vi "ExecuteSkill.vi"(0 "object in":refnum<class "GoToTargetPositionSkill.lvclass">, 2 "Robot in":refnum<class "Robot.lvclass">, 4 "GameRef":refnum<data-value>, 5 "error in (no error)":errorcluster) -> (14 "object out":refnum<class "GoToTargetPositionSkill.lvclass">, 16 "Robot out":refnum<class "Robot.lvclass">, 19 "error out":errorcluster)   [LabVIEW 2023, in "GoToTargetPositionSkill.lvclass"]
uses:
  GoToTargetPositionSkill.lvclass
  Robot_class/Robot.lvclass
  Game_class/Game.lvclass
  Ball_class/Ball.lvclass
  Zone_class/Zone.lvclass
  GoToSkill_v2_class/GoToSkill_v2.lvclass
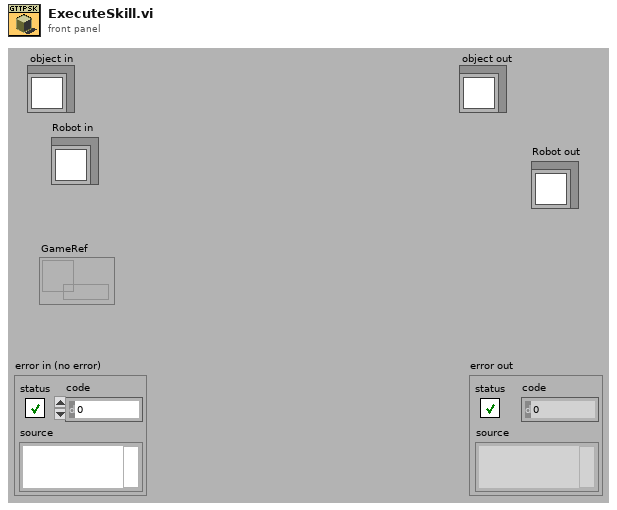
[diagram p1: front panel]
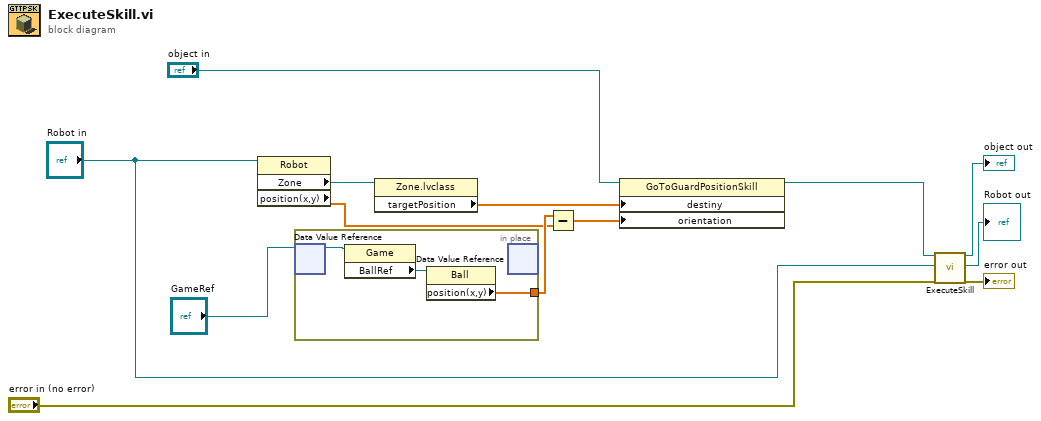
[diagram p0: block diagram]
diagram:
  n1 = property class="Robot"(reference="Robot in") -> ("Zone"=w6:refnum<class "Zone.lvclass">, "position(x,y)"=w1:dbl[])  [unwired: 1 in, 2 out]
  n2 = in-place {
    in-place-border: [w14] -> w2
    n3 = in-place-dvr #1("GameRef") -> (w16:refnum<class "Game.lvclass">)  [unwired: 1 out]
    n4 = property class="Game"(reference=w16) -> ("BallRef"=w15:refnum<class "Ball.lvclass">)  [unwired: 1 in, 2 out]
    n5 = property class="Ball"(reference=w15) -> ("position(x,y)"=w14:dbl[])  [unwired: 1 in, 2 out]
    n6 = in-place-dvr #1() -> ()  [unwired: 1 in, 2 out]
  }
  n7 = property class="Zone.lvclass"(reference=w6) -> ("targetPosition"=w5:dbl[])  [unwired: 1 in, 2 out]
  n8 = Subtract(x=w2, y=w1) -> (x-y=w7:dbl[])
  n9 = property class="GoToGuardPositionSkill"(reference="object in", "destiny"=w5, "orientation"=w7) -> (reference out=w4:refnum<class "GoToTargetPositionSkill.lvclass">)  [unwired: 1 in, 1 out]
  n10 = call-parent "ExecuteSkill.vi"("object in"=w4, "Robot in"="Robot in", "error in (no error)"="error in (no error)") -> ("object out"=→"object out":refnum<class "GoToTargetPositionSkill.lvclass">, "Robot out"=→"Robot out":refnum<class "Robot.lvclass">, "error out"=→"error out":errorcluster)  [unwired: 14 in]
